vi "stop_all_test.vi"(8 "error in (no error)":errorcluster, 9 "Message Queues in":T2, 11 "test mode":T1(ring)) -> (0 "error out":errorcluster)   [LabVIEW 2015]
uses:
  support/Message Queue/All Message Queues.ctl
  support/Message Queue/Message Cluster.ctl
  support/Message Queue/Enqueue Message (Single).vi
  support/Message Queue/Message Queue.lvlib
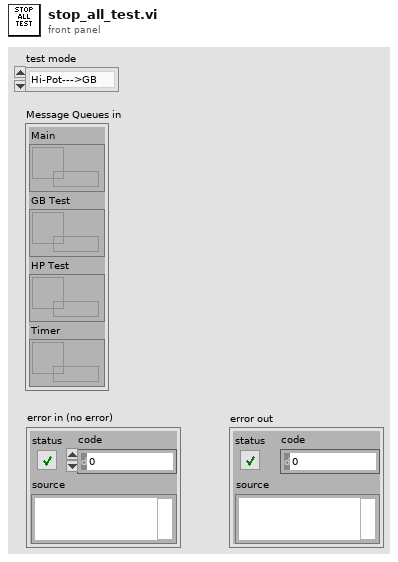
[diagram p1: front panel]
types:
  T1 = enum16{"Hi-Pot--->GB", "GB--->Hi-Pot", "Hi-Pot only", "GB only"}
  T2 = typedef "Message Queue.lvlib/All Message Queues.ctl" = cluster{"Main":refnum<queue>, "GB Test":refnum<queue>, "HP Test":refnum<queue>, "Timer":refnum<queue>}
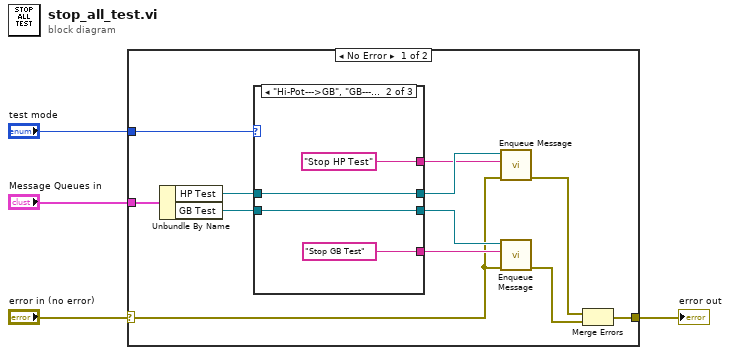
[diagram p0: block diagram]
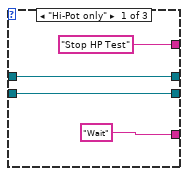
[diagram p2: hidden frame]
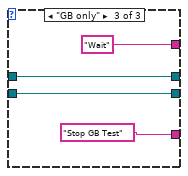
[diagram p3: hidden frame]
diagram:
  n1 = case shown="No Error" "error in (no error)" {
    selector: "error in (no error)" -> [w5 w29]
    tunnel: "Message Queues in" -> [w14 _]
    tunnel: "test mode" -> [w11 _]
    tunnel: [w7 w29] -> w2
    frame No Error {
      n2 = Unbundle By Name(w14) -> ("HP Test"=w15:refnum<queue>, "GB Test"=w16:refnum<queue>)
      n3 = case shown="\"Hi-Pot--->GB\", \"GB--->Hi-Pot\"" w11 {
        tunnel: w15 -> [w19 w24 w28]
        tunnel: [w19 w24 w28] -> w9
        tunnel: w16 -> [w18 w23 w27]
        tunnel: [w18 w23 w27] -> w10
        tunnel: ["Wait" "Stop GB Test" "Stop GB Test"] -> w12
        tunnel: ["Stop HP Test" "Stop HP Test" "Wait"] -> w8
        frame "Hi-Pot only" {
        }
        frame "Hi-Pot--->GB", "GB--->Hi-Pot" {
        }
        frame "GB only" {
        }
      }
      n4 = call-poly "Enqueue Message.vi"("error in (no error)"=w5, "Message"=w8, "Message Queue"=w9) -> ("error out"=w13:errorcluster)  [unwired: 7 in, 1 out]
      n5 = call-poly "Enqueue Message.vi"("error in (no error)"=w5, "Message"=w12, "Message Queue"=w10) -> ("error out"=w6:errorcluster)  [unwired: 7 in, 1 out]
      n6 = Merge Errors(w13, w6) -> (w7:errorcluster)
    }
    frame Error {
    }
  }
  "error out" <- w2
